vi "Year2019 Q4.vi"() -> ()   [LabVIEW 2018]
panel:
  out "Tip Amount":dbl
  in  "Service":bool
  in  "Food":bool
  in  "stop":bool
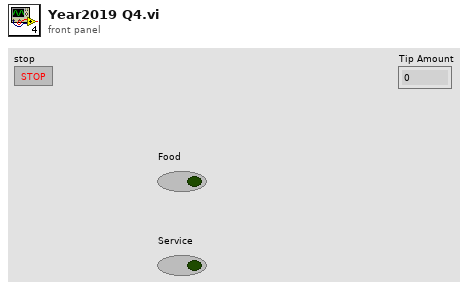
[diagram p1: front panel]
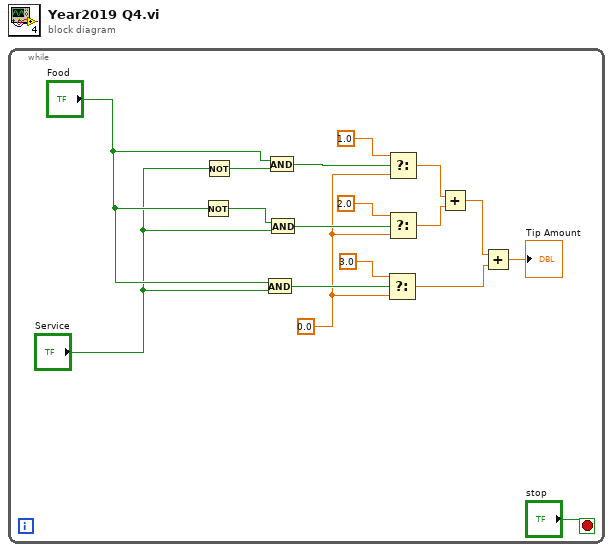
[diagram p0: block diagram]
diagram:
  n1 = while {
    stop <- "stop" stop-if-true
    w9 = 0.0 ("f")
    n2 = Not(x="Food") -> (.not. x?=w15:bool)
    n3 = Not(x="Service") -> (.not. x?=w16:bool)
    n4 = And(x="Food", y="Service") -> (x .and. y?=w10:bool)
    n5 = And(x="Food", y=w16) -> (x .and. y?=w12:bool)
    n6 = And(x=w15, y="Service") -> (x .and. y?=w11:bool)
    n7 = Select(t=3.0, s=w10, f=w9) -> (s? t:f=w2:dbl)
    n8 = Select(t=1.0, s=w12, f=w9) -> (s? t:f=w4:dbl)
    n9 = Select(t=2.0, s=w11, f=w9) -> (s? t:f=w5:dbl)
    n10 = Add(x=w4, y=w5) -> (x+y=w3:dbl)
    n11 = Add(x=w3, y=w2) -> (x+y=→"Tip Amount":dbl)
  }
